vi "Drop default VCluster data.vi"(7 "Drop default numeric? (F)":bool, 8 "error in (no error)":errorcluster, 10 "Columns":string[](array[string]), 11 "VCluster in":variant) -> (0 "error out":errorcluster, 2 "VCluster Columns":string[](array[string]), 3 "VCluster out":variant)   [LabVIEW 2020, in "Database Reuse.lvlib"]
uses:
  Database Reuse.lvlib
  <vilib>/Utility/Data Type/NI_Data Type.lvlib
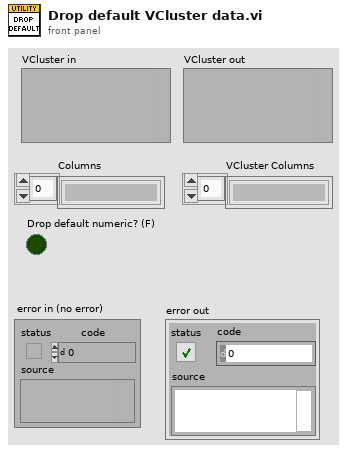
[diagram p1: front panel]
types:
  T1 = typedef "NI_Data Type.lvlib/Data Type.ctl" = enum8{"Invalid Type", "Void", "I8", "I16", "I32", "I64", "U8", "U16", "U32", "U64", "Single Float", "Double Float", "Extended Float", "Single Complex", "Double Complex", "Extended Complex", "Enum U8", "Enum U16", "Enum U32", "Enum U64", "Single Float With Unit", "Double Float With Unit", "Extended Float With Unit", "Single Complex with Unit", "Double Complex with Unit", "Extended Complex with Unit", "Boolean", "String", "Path", "Picture", "Tag", "Array", "Cluster", "Variant", "LV Variant", "Waveform", "Timestamp", "Digital Waveform", "Digital Data", "ExpressData", "Refnum", "External Data", "VI", "Poly VI", "LabVIEW Class Instance", "Fixed Point", "Set Collection", "Map Collection"}
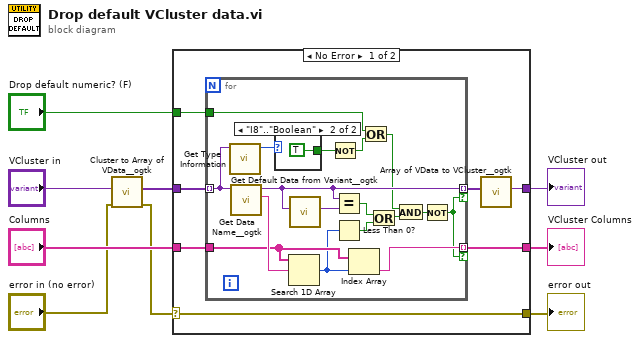
[diagram p0: block diagram]
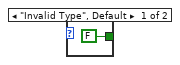
[diagram p2: hidden frame]
diagram:
  n1 = call <userlib>:"Cluster to Array of VData__ogtk.vi"("error in (no error)"="error in (no error)", "Cluster"="VCluster in") -> ("error out"=w1:errorcluster, "Array of VData"=w4:variant[])  [unwired: 8 in]
  n2 = case shown="No Error" w1 {
    selector: w1 -> [w12 w36]
    tunnel: "Drop default numeric? (F)" -> [w16 _]
    tunnel: [w15 _] -> w8
    tunnel: "Columns" -> [w14 _]
    tunnel: w4 -> [w13 _]
    tunnel: [w12 w36] -> w6
    tunnel: [w10 _] -> w5
    frame No Error {
      n3 = for {
        tunnel: w13 -> [w25] mode=indexing
        tunnel: w14 -> [w32]
        tunnel: [w30] -> w11 mode=indexing if=w17
        tunnel: [w28] -> w15 mode=indexing if=w17
        tunnel: w16 -> [w21]
        n4 = call <vilib>:"Get Type Information.vi"("variant"=w25) -> ("type"=w24:T1)  [unwired: 6 in, 4 out]
        n5 = call <userlib>:"Get Data Name__ogtk.vi"("Data"=w25) -> ("Data Name"=w33:string, "Data dup"=w30:variant)  [unwired: 8 in, 1 out]
        n6 = case shown="\"I8\"..\"Boolean\"" w24 {
          tunnel: [FALSE TRUE] -> w20
          frame "Invalid Type", Default {
          }
          frame "I8".."Boolean" {
          }
        }
        n7 = Search 1D Array(1D array=w32, element=w33) -> (index of element=w31:i32)  [unwired: 1 in]
        n8 = call <userlib>:"Get Default Data from Variant__ogtk.vi"("Variant"=w30) -> ("Default VData"=w29:variant)  [unwired: 9 in, 1 out]
        n9 = Not(x=w20) -> (.not. x?=w19:bool)
        n10 = Equal?(x=w30, y=w29) -> (x = y?=w26:bool)
        n11 = Less Than 0?(x=w31) -> (x < 0?=w27:bool)
        n12 = Index Array(array=w32, index=w31) -> (element=w28:string)
        n13 = Or(x=w21, y=w19) -> (x .or. y?=w22:bool)
        n14 = Or(x=w26, y=w27) -> (x .or. y?=w23:bool)
        n15 = And(x=w22, y=w23) -> (x .and. y?=w18:bool)
        n16 = Not(x=w18) -> (.not. x?=w17:bool)
      }
      n17 = call <userlib>:"Array of VData to VCluster__ogtk.vi"("Array"=w11) -> ("VCluster"=w10:variant)  [unwired: 9 in, 1 out]
    }
    frame Error {
    }
  }
  "VCluster out" <- w5
  "VCluster Columns" <- w8
  "error out" <- w6
